vi "CreateSelfReference.vi"(8 "error in (no error)":errorcluster, 11 "Analyzer":refnum<class "Analyzer.lvclass">) -> (0 "error out":errorcluster, 3 "Analyzer out":refnum<class "Analyzer.lvclass">)   [LabVIEW 2022 SP3, in "Analyzer.lvclass"]
uses:
  Analyzer.lvclass
  Analyzer.lvclass/Analyzer.ctl
  <vilib>/JKI/JKI SMO/SMO/SMO.lvclass
panel:
  # "For instructions on how to use the JKI State Machine Objects, examples and video tutorials, visit:\nhttp://jki.net/state-machine-objects/\n\nJKI State Machine Objects™\nhttp://jki.net/state-machine-objects/\nCopyright (C) 2005-2015, JKI <info@jki.net>\nALL RIGHTS RESERVED"
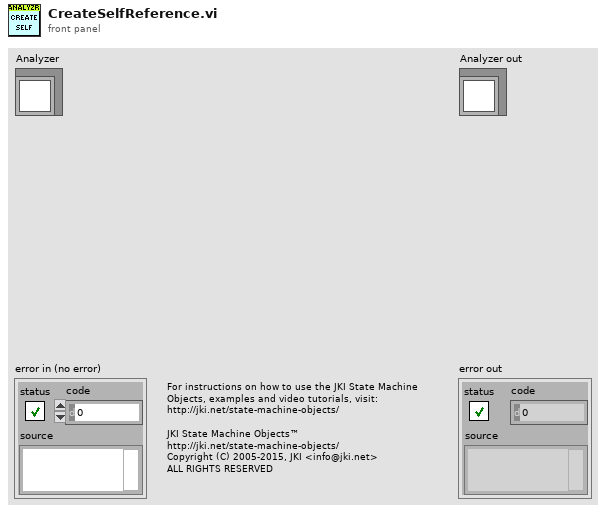
[diagram p1: front panel]
types:
  T1 = typedef "Analyzer.lvclass/PrivateData--Ref.ctl" = refnum<data-value>
  T2 = typedef "Analyzer.lvclass/PrivateData--Cluster.ctl" = cluster{"Public Events":T3, "Subpanel Ref":refnum<vi>, "UI State":T4, "Private Events":T5}
  T3 = typedef "Analyzer.lvclass/PublicEvents--Cluster.ctl" = cluster{"UI State":refnum<user-event>, "NewEventMessage":refnum<user-event>}
  T4 = typedef "Analyzer.lvclass/Analyzer State--enum.ctl" = enum16{"unknown", "Opened", "Embedded", "Closed"}
  T5 = typedef "Analyzer.lvclass/PrivateEvents--Cluster.ctl" = cluster{"NewRequest":refnum<user-event>}
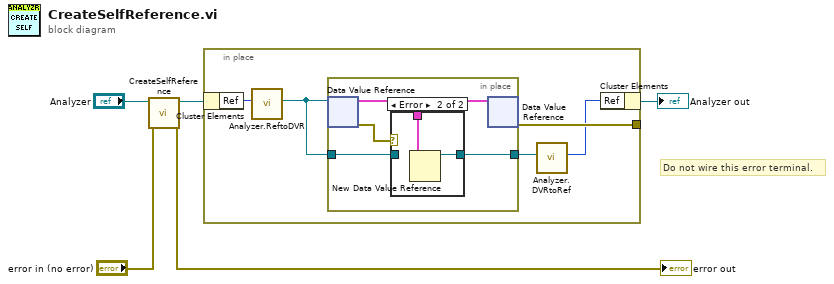
[diagram p0: block diagram]
diagram:
  # "Do not wire this error terminal."
  n1 = call-parent "CreateSelfReference.vi"("error in (no error)"="error in (no error)", "SMO"="Analyzer") -> ("error out"=→"error out":errorcluster, "SMO out"=w3:refnum<class "Analyzer.lvclass">)  [unwired: 8 in]
  n2 = in-place {
    in-place-border: [w10] -> _
    n3 = in-place-cluster #1(w3) -> ("Ref"=w9:u32)
    n4 = call "Analyzer.ReftoDVR.vi"("Ref"=w9) -> ("Ref"=w8:T1)  [unwired: 10 in]
    n5 = in-place {
      in-place-border: [w14] -> w7
      in-place-border: w8 -> [w11]
      n6 = in-place-dvr #2(w8) -> (w13:T2, w12:errorcluster)
      n7 = case shown="Error" w12 {
        tunnel: [w15 w17] -> w14
        tunnel: w13 -> [_ w16]
        tunnel: w11 -> [w15 _]
        frame No Error {
        }
        frame Error {
          n8 = New Data Value Reference(data value=w16) -> (data value reference=w17:refnum<data-value>)  [unwired: 1 in, 1 out]
        }
      }
      n9 = in-place-dvr #2(w13) -> (w10:errorcluster)  [unwired: 1 out]
    }
    n10 = call "Analyzer.DVRtoRef.vi"("Ref"=w7) -> ("Ref"=w6:u32)  [unwired: 10 in]
    n11 = in-place-cluster #1("Ref"=w6) -> (→"Analyzer out":refnum<class "Analyzer.lvclass">)
  }
